vi "Rotate Waypoints Pre.vi"(9 "Pt 2":cluster{"x":dbl, "y":dbl, "th":dbl}, 10 "Pt 1":cluster{"x":dbl, "y":dbl, "th":dbl}, 11 "Pt 0":cluster{"x":dbl, "y":dbl, "th":dbl}) -> (1 "Pt 2 out":cluster{dbl, dbl, dbl}, 2 "Pt 1 out":cluster{"Vertex Dist":dbl, dbl, dbl}, 3 "Pt 1 rel to Pt0":cluster{"Vertex Dist":dbl, dbl, dbl})   [LabVIEW 2025]
panel:
  out "XY Graph":cluster{cluster{"x":dbl, "y":dbl}[]}[](graph)
  # "White plot is three input waypts\nred plot is at origin and rotated so\nfirst segment is at 0deg\nthird plot is pt1 rotated to be at 0deg, \nbut offset from original pt0"
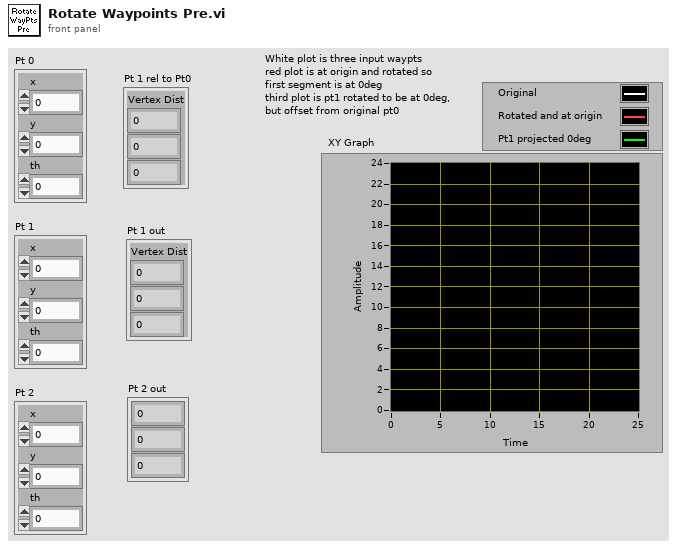
[diagram p1: front panel]
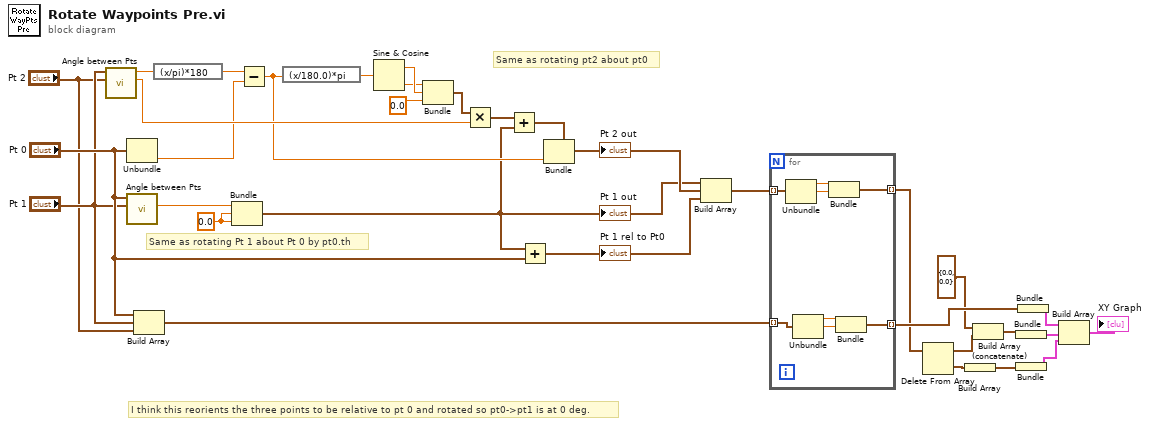
[diagram p0: block diagram]
diagram:
  w24 = 0.0
  # "I think this reorients the three points to be relative to pt 0 and rotated so pt0->pt1 is at 0 deg."
  # "Same as rotating pt2 about pt0"
  # "Same as rotating Pt 1 about Pt 0 by pt0.th"
  n1 = call "Angle between Pts.vi"("Pt 2"="Pt 2", "Pt 1"="Pt 1") -> ("Distance ft"=w29:dbl, "Angle rad"=w26:dbl)  [unwired: 8 in]
  n2 = Unbundle("Pt 0") -> ("th"=w23:dbl)  [unwired: 2 out]
  n3 = call "Angle between Pts.vi"("Pt 2"="Pt 1", "Pt 1"="Pt 0") -> ("Distance ft"=w20:dbl)  [unwired: 8 in, 1 out]
  n4 = Build Array("Pt 0", "Pt 1", "Pt 2") -> (w16:cluster{"x":dbl, "y":dbl, "th":dbl}[])
  n5 = expression code="(x/pi)*180" ("radians to degrees")(w26) -> (w25:dbl)
  n6 = Bundle("Distance ft"=w20, w24, w24) -> (w1:cluster{"Distance ft":dbl, dbl, dbl})  [unwired: 1 in]
  "Pt 1 out" <- w1
  n7 = Subtract(x=w25, y=w23) -> (x-y=w27:dbl)
  n8 = expression code="(x/180.0)*pi" ("degrees to radians")(w27) -> (w33:dbl)
  n9 = Sine & Cosine(0:w33) -> (1:w32:dbl, 2:w31:dbl)
  n10 = Bundle(w31, w32, 0.0) -> (w30:cluster{dbl, dbl, dbl})  [unwired: 1 in]
  n11 = Multiply(x=w30, y=w29) -> (x*y=w22:cluster{dbl, dbl, dbl})
  n12 = Add(x=w22, y=w1) -> (x+y=w21:cluster{dbl, dbl, dbl})
  n13 = Add(x=w1, y="Pt 0") -> (x+y=w15:cluster{dbl, dbl, dbl})
  "Pt 1 rel to Pt0" <- w15
  n14 = Bundle(cluster=w21, w27) -> (w2:cluster{dbl, dbl, dbl})  [unwired: 2 in]
  "Pt 2 out" <- w2
  n15 = Build Array(w1, w2, w15) -> (w14:cluster{"Distance ft":dbl, dbl, dbl}[])
  n16 = for {
    tunnel: w16 -> [w41] mode=indexing
    tunnel: [w38] -> w11 mode=indexing
    tunnel: w14 -> [w35] mode=indexing
    tunnel: [w34] -> w8 mode=indexing
    n17 = Unbundle(w35) -> ("Distance ft"=w36:dbl, w37:dbl)  [unwired: 1 out]
    n18 = Unbundle(w41) -> ("x"=w40:dbl, "y"=w39:dbl)  [unwired: 1 out]
    n19 = Bundle("Distance ft"=w36, w37) -> (w34:cluster{"Distance ft":dbl, dbl})  [unwired: 1 in]
    n20 = Bundle("x"=w40, "y"=w39) -> (w38:cluster{"x":dbl, "y":dbl})  [unwired: 1 in]
  }
  n21 = Delete From Array(array=w8) -> (deleted portion=w7:cluster{"Distance ft":dbl, dbl}, array with subset deleted=w5:cluster{"Distance ft":dbl, dbl}[])  [unwired: 2 in]
  n22 = Build Array(w7) -> (w6:cluster{"Distance ft":dbl, dbl}[])
  n23 = Build Array (concatenate)(cluster{"Distance ft":dbl, dbl} {"Distance ft"=0.0, 0.0} ("deleted portion"), w5) -> (w4:cluster{"Distance ft":dbl, dbl}[])
  n24 = Bundle(w4) -> (w10:cluster{cluster{"Distance ft":dbl, dbl}[]})  [unwired: 1 in]
  n25 = Bundle(w6) -> (w9:cluster{cluster{"Distance ft":dbl, dbl}[]})  [unwired: 1 in]
  n26 = Bundle(w11) -> (w12:cluster{cluster{"x":dbl, "y":dbl}[]})  [unwired: 1 in]
  n27 = Build Array(w12, w10, w9) -> (→"XY Graph":cluster{cluster{"Distance ft":dbl, "y":dbl}[]}[])
